vi "VersionStrings.GetVeristandStepsProjectPath.vi"(1 "Workspace Path":string) -> (0 "VeristandSteps.csproj File Path":string)   [LabVIEW 2014, in "VeriStand Steps Version Mutation.lvlib"]
uses:
  VeriStand Steps Version Mutation.lvlib
  Types/Constants.vi
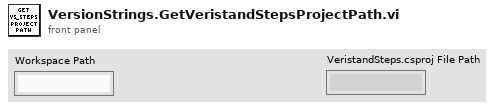
[diagram p1: front panel]
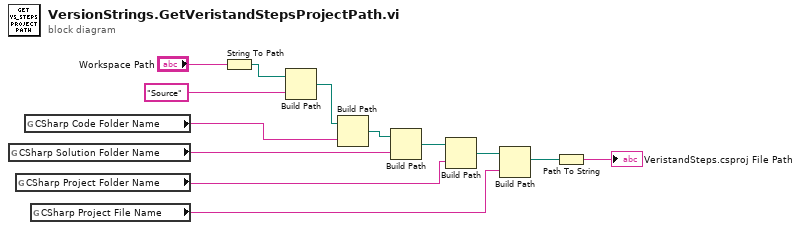
[diagram p0: block diagram]
diagram:
  n1 = global read "Constants.vi" "CSharp Solution Folder Name"() -> (w3:string)
  n2 = global read "Constants.vi" "CSharp Project Folder Name"() -> (w2:string)
  n3 = global read "Constants.vi" "CSharp Code Folder Name"() -> (w4:string)
  n4 = global read "Constants.vi" "CSharp Project File Name"() -> (w1:string)
  n5 = String To Path(string="Workspace Path") -> (path=w8:path)
  n6 = Build Path(base path=w8, name or relative path="Source") -> (appended path=w7:path)
  n7 = Build Path(base path=w7, name or relative path=w4) -> (appended path=w11:path)
  n8 = Build Path(base path=w11, name or relative path=w3) -> (appended path=w12:path)
  n9 = Build Path(base path=w12, name or relative path=w2) -> (appended path=w13:path)
  n10 = Build Path(base path=w13, name or relative path=w1) -> (appended path=w5:path)
  n11 = Path To String(path=w5) -> (string=→"VeristandSteps.csproj File Path":string)
